vi "day 11 task 2.vi"() -> ()   [LabVIEW 2019]
uses:
  <userlib>/_OpenG.lib/array/array.llb/Search 1D Array (I32)__ogtk.vi
panel:
  out "Monkeys":T1(array[cluster])
  out "Array":T1(array[cluster])
  out "level of monkey business":u64
  out "Amount of inspections by each monkey":u64[](array[numeric])
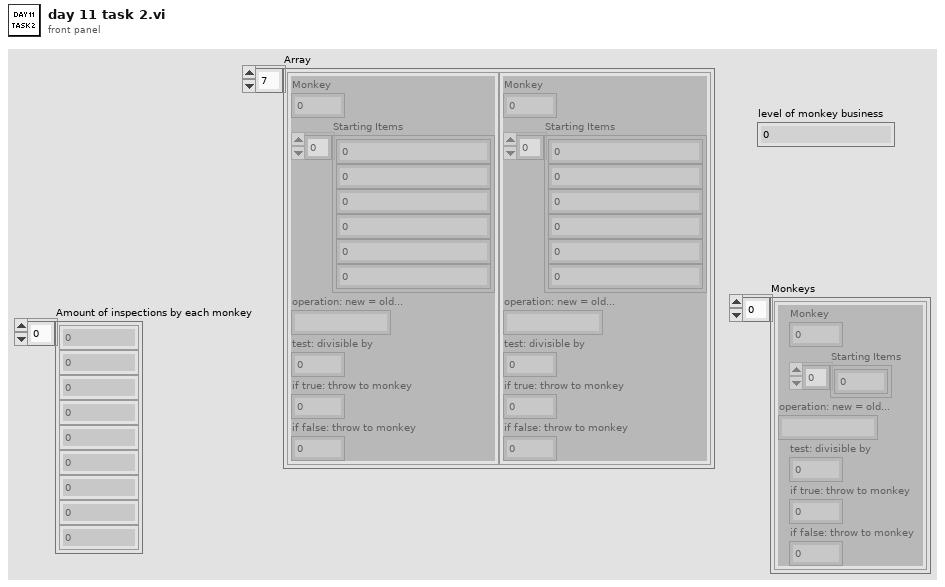
[diagram p1: front panel]
types:
  T1 = cluster{"Monkey":i32, "Starting Items":u64[], "operation: new = old...":string, "test: divisible by":u64, "if true: throw to monkey":i32, "if false: throw to monkey":i32}[]
  T2 = cluster{"Monkey":i32, "Starting Items":u64[], "operation: new = old...":string, "test: divisible by":u64, "if true: throw to monkey":i32, "if false: throw to monkey":i32}
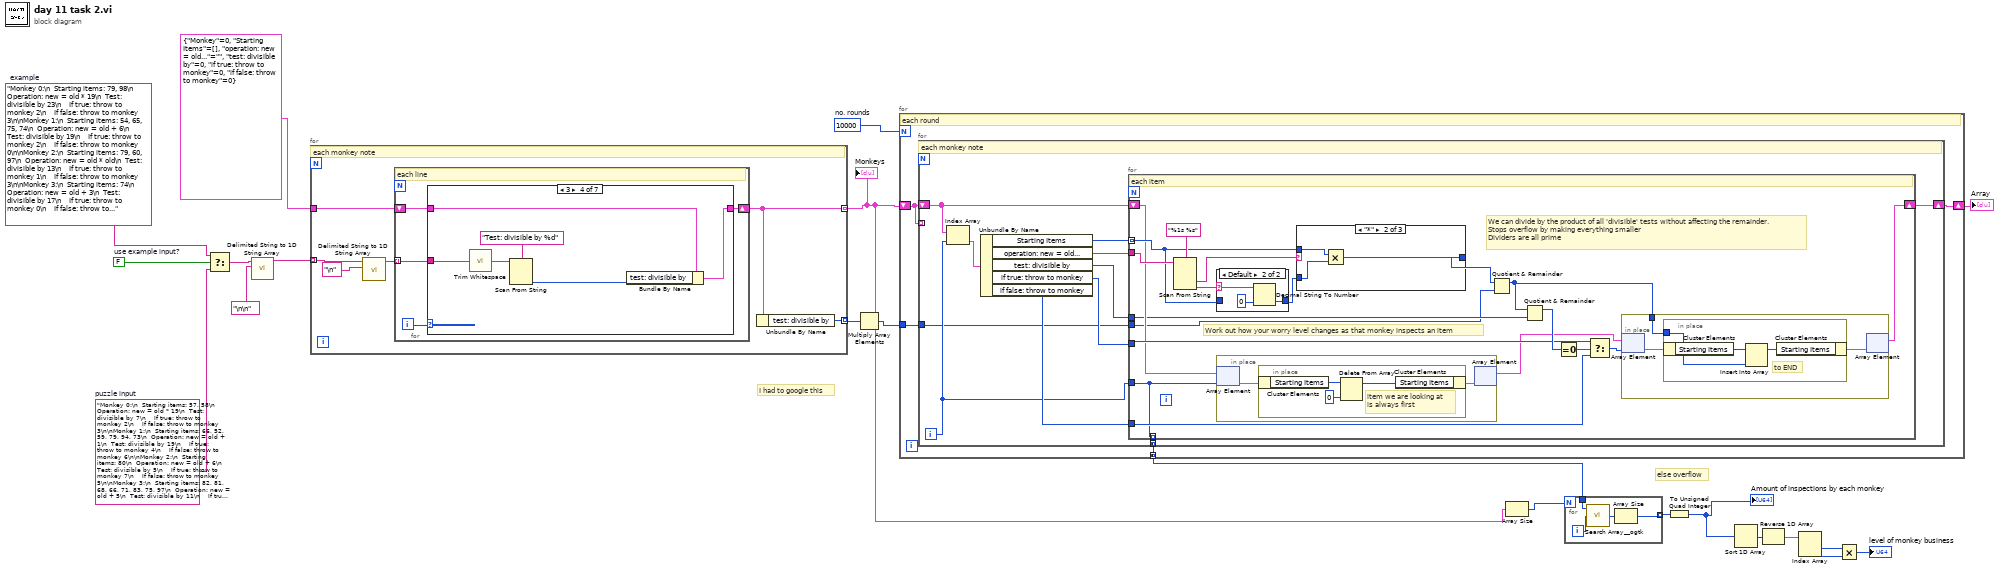
[diagram p0: block diagram]
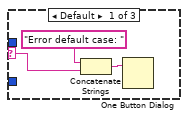
[diagram p3: hidden frame]
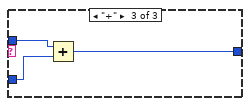
[diagram p4: hidden frame]
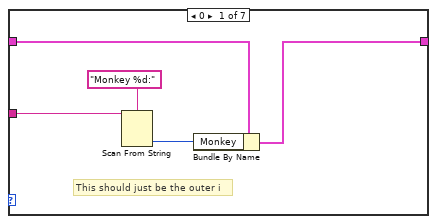
[diagram p5: hidden frame]
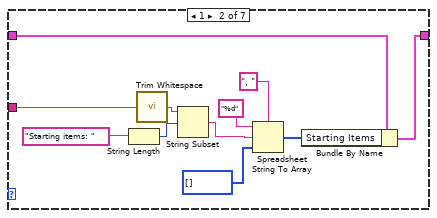
[diagram p6: hidden frame]
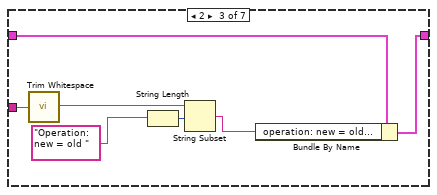
[diagram p7: hidden frame]
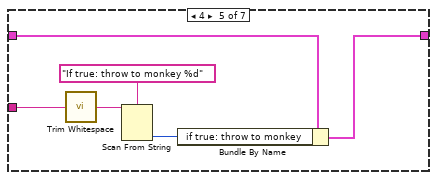
[diagram p8: hidden frame]
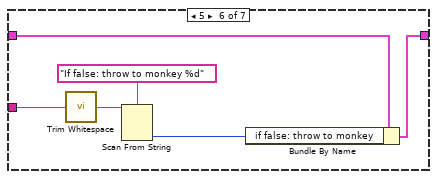
[diagram p9: hidden frame]
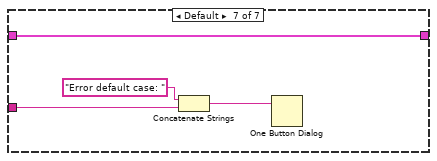
[diagram p10: hidden frame]
diagram:
  w14 = 10000  # no. rounds
  w19 = "Monkey 0:\n  Starting items: 79, 98\n  Operation: new = old * 19\n  Test: divisible by 23\n    If true: throw to monkey 2\n    If false: throw to monkey 3\n\nMonkey 1:\n  Starting items: 54, 65, 75, 74\n  Operation: new = old + 6\n  Test: divisible by 19\n    If true: throw to monkey 2\n    If false: throw to monkey 0\n\nMonkey 2:\n  Starting items: 79, 60, 97\n  Operation: new = old * old\n  Test: divisible by 13\n    If true: throw to monkey 1\n    If false: throw to monkey 3\n\nMonkey 3:\n  Starting items: 74\n  Operation: new = old + 3\n  Test: divisible by 17\n    If true: throw to monkey 0\n    If false: throw to monkey 1"  # example
  w20 = FALSE  # use example input?
  w21 = "Monkey 0:\n  Starting items: 57, 58\n  Operation: new = old * 19\n  Test: divisible by 7\n    If true: throw to monkey 2\n    If false: throw to monkey 3\n\nMonkey 1:\n  Starting items: 66, 52, 59, 79, 94, 73\n  Operation: new = old + 1\n  Test: divisible by 19\n    If true: throw to monkey 4\n    If false: throw to monkey 6\n\nMonkey 2:\n  Starting items: 80\n  Operation: new = old + 6\n  Test: divisible by 5\n    If true: throw to monkey 7\n    If false: throw to monkey 5\n\nMonkey 3:\n  Starting items: 82, 81, 68, 66, 71, 83, 75, 97\n  Operation: new = old + 5\n  Test: divisible by 11\n    If true: throw to monkey 5\n    If false: throw to monkey 2\n\nMonkey 4:\n  Starting items: 55, 52, 67, 70, 69, 94, 90\n  Operation: new = old * old\n  Test: divisible by 17\n    If true: throw to monkey 0\n    If false: throw to monkey 3\n\nMonkey 5:\n  Starting items: 69, 85, 89, 91\n  Operation: new = old + 7\n  Test: divisible by 13\n    If true: throw to monkey 1\n    If false: throw to monkey 7\n\nMonkey 6:\n  Starting items: 75, 53, 73, 52, 75\n  Operation: new = old * 7\n  Test: divisible by 2\n    If true: throw to monkey 0\n    If false: throw to monkey 4\n\nMonkey 7:\n  Starting items: 94, 60, 79\n  Operation: new = old + 2\n  Test: divisible by 3\n    If true: throw to monkey 1\n    If false: throw to monkey 6"  # puzzle input
  # "else overflow"
  # "I had to google this"
  n1 = Select(t=w19, s=w20, f=w21) -> (s? t:f=w18:string)
  n2 = call <vilib>:"Delimited String to 1D String Array.vi"("delimiter"="\n\n" ("regular expression"), "delimited string"=w18) -> ("string array"=w16:string[])  [unwired: 9 in]
  n3 = for {
    tunnel: w16 -> [w27] mode=indexing
    tunnel: T2 {"Monkey"=0, "Starting Items"=[], "operation: new = old..."="", "test: divisible by"=0, "if true: throw to monkey"=0, "if false: throw to monkey"=0} -> [w26]
    tunnel: [w23] -> w12 mode=indexing
    tunnel: [w22] -> w4 mode=indexing
    # "each monkey note"
    n4 = call <vilib>:"Delimited String to 1D String Array.vi"("delimiter"="\n", "delimited string"=w27) -> ("string array"=w25:string[])  [unwired: 9 in]
    n5 = for {
      tunnel: w25 -> [w30] mode=indexing
      shift-right: [w29] -> w23
      shift-left: w26 -> [w28]
      i -> [w31]
      # "each line"
      n6 = case shown="3" w31 {
        tunnel: w30 -> [w36 w44 w54 w58 w64 w70 w74]
        tunnel: [w34 w41 w52 w55 w61 w67 w73] -> w29
        tunnel: w28 -> [w33 w42 w53 w56 w62 w69 w73]
        frame 0 {
          # "This should just be the outer i"
          n7 = Scan From String(format string="Monkey %d:", input string=w36) -> (output 1=w32:i32)  [unwired: 3 in, 3 out]
          n8 = Bundle By Name(cluster=w33, "Monkey"=w32) -> (w34:T2)
        }
        frame 1 {
          n9 = String Length(string="Starting items: " ("format string")) -> (length=w38:i32)
          n10 = call <vilib>:"Trim Whitespace.vi"("string"=w44) -> ("trimmed string"=w37:string)  [unwired: 1 in]
          n11 = String Subset(string=w37, offset (0)=w38) -> (substring=w40:string)  [unwired: 1 in]
          n12 = Spreadsheet String To Array(delimiter (Tab)=", ", format string="%d", spreadsheet string=w40, array type (2D Dbl)=u64[] []) -> (array=w43:u64[])
          n13 = Bundle By Name(cluster=w42, "Starting Items"=w43) -> (w41:T2)
        }
        frame 2 {
          n14 = call <vilib>:"Trim Whitespace.vi"("string"=w54) -> ("trimmed string"=w50:string)  [unwired: 1 in]
          n15 = String Length(string="Operation: new = old " ("format string")) -> (length=w48:i32)
          n16 = String Subset(string=w50, offset (0)=w48) -> (substring=w51:string)  [unwired: 1 in]
          n17 = Bundle By Name(cluster=w53, "operation: new = old..."=w51) -> (w52:T2)
        }
        frame 3 {
          n18 = call <vilib>:"Trim Whitespace.vi"("string"=w58) -> ("trimmed string"=w59:string)  [unwired: 1 in]
          n19 = Scan From String(format string="Test: divisible by %d", input string=w59) -> (output 1=w57:i32)  [unwired: 3 in, 3 out]
          n20 = Bundle By Name(cluster=w56, "test: divisible by"=w57) -> (w55:T2)
        }
        frame 4 {
          n21 = call <vilib>:"Trim Whitespace.vi"("string"=w64) -> ("trimmed string"=w65:string)  [unwired: 1 in]
          n22 = Scan From String(format string="If true: throw to monkey %d", input string=w65) -> (output 1=w63:i32)  [unwired: 3 in, 3 out]
          n23 = Bundle By Name(cluster=w62, "if true: throw to monkey"=w63) -> (w61:T2)
        }
        frame 5 {
          n24 = call <vilib>:"Trim Whitespace.vi"("string"=w70) -> ("trimmed string"=w71:string)  [unwired: 1 in]
          n25 = Scan From String(format string="If false: throw to monkey %d", input string=w71) -> (output 1=w68:i32)  [unwired: 3 in, 3 out]
          n26 = Bundle By Name(cluster=w69, "if false: throw to monkey"=w68) -> (w67:T2)
        }
        frame Default {
          n27 = Concatenate Strings("Error default case: " ("message"), w74) -> (w75:string)
          n28 = One Button Dialog(message=w75) -> ()  [unwired: 1 in, 1 out]
        }
      }
    }
    n29 = Unbundle By Name(w23) -> ("test: divisible by"=w22:u64)
  }
  "Monkeys" <- w12
  n30 = Multiply Array Elements(1:w4) -> (0:w3:u64)
  n31 = for {
    N: w14 -> [_]
    shift-right: [w80] -> w5
    shift-left: w12 -> [w79]
    tunnel: [w78] -> w11 mode=concatenating
    tunnel: w3 -> [w77]
    # "each round"
    n32 = for {
      shift-right: [w87] -> w80
      shift-left: w79 -> [w86]
      tunnel: w79 -> [_] mode=indexing
      tunnel: [w82] -> w78 mode=concatenating
      tunnel: w77 -> [w81]
      i -> [w83]
      # "each monkey note"
      n33 = Index Array(array=w86, index=w83) -> (element=w90:T2)
      n34 = Unbundle By Name(w90) -> ("Starting Items"=w91:u64[], "operation: new = old..."=w89:string, "test: divisible by"=w88:u64, "if true: throw to monkey"=w85:i32, "if false: throw to monkey"=w84:i32)
      n35 = for {
        tunnel: w91 -> [w105] mode=indexing
        tunnel: w89 -> [w110]
        tunnel: w88 -> [w95]
        shift-right: [w97] -> w87
        shift-left: w86 -> [w99]
        tunnel: w85 -> [w102]
        tunnel: w84 -> [w101]
        tunnel: w83 -> [w96]
        tunnel: [w96] -> w82 mode=indexing
        tunnel: w81 -> [w93]
        # "We can divide by the product of all 'divisible' tests without affecting the remainder.\nStops overflow by making everything smaller\nDividers are all prime"
        # "Work out how your worry level changes as that monkey inspects an item"
        # "each item"
        n36 = Scan From String(format string="%1s %s", input string=w110) -> (output 1=w108:string, output 2=w107:string)  [unwired: 4 in, 3 out]
        n37 = case shown="Default" w107 {
          selector: w107 -> [_ w125]
          tunnel: [w122 w124] -> w106
          tunnel: w105 -> [w122 _]
          frame "old" {
          }
          frame Default {
            n38 = Decimal String To Number(string=w125, default (0L)=u64 0) -> (number=w124:u64)  [unwired: 1 in, 1 out]
          }
        }
        n39 = in-place {
          n40 = in-place-array #1(w99, w96) -> (w118:T2)
          n41 = in-place {
            # "item we are looking at \nis always first"
            n42 = in-place-cluster #2(w118) -> ("Starting Items"=w120:u64[])
            n43 = Delete From Array(array=w120, index=0) -> (array with subset deleted=w121:u64[])  [unwired: 1 in, 1 out]
            n44 = in-place-cluster #2("Starting Items"=w121) -> (w117:T2)
          }
          n45 = in-place-array #1(w117) -> (w98:T1)  [unwired: 1 out]
        }
        n46 = case shown="\"*\"" w108 {
          selector: w108 -> [w126 _ _]
          tunnel: w106 -> [_ w130 w134]
          tunnel: w105 -> [_ w131 w133]
          tunnel: [_ w129 w132] -> w94
          frame Default {
            n47 = Concatenate Strings("Error default case: " ("message"), w126) -> (w128:string)
            n48 = One Button Dialog(message=w128) -> ()  [unwired: 1 in, 1 out]
          }
          frame "*" {
            n49 = Multiply(x=w131, y=w130) -> (x*y=w129:u64)
          }
          frame "+" {
            n50 = Add(x=w133, y=w134) -> (x+y=w132:u64)
          }
        }
        n51 = Quotient & Remainder(x=w94, y=w93) -> (x-y*floor(x/y)=w92:u64)  [unwired: 1 out]
        n52 = Quotient & Remainder(x=w92, y=w95) -> (x-y*floor(x/y)=w104:u64)  [unwired: 1 out]
        n53 = Equal To 0?(x=w104) -> (x = 0?=w103:bool)
        n54 = Select(t=w102, s=w103, f=w101) -> (s? t:f=w100:i32)
        n55 = in-place {
          in-place-border: w92 -> [w113]
          n56 = in-place-array #3(w98, w100) -> (w111:T2)
          n57 = in-place {
            in-place-border: w113 -> [w115]
            # "to END"
            n58 = in-place-cluster #4(w111) -> ("Starting Items"=w114:u64[])
            n59 = Insert Into Array(array=w114, new element=w115) -> (w116:u64[])  [unwired: 1 in]
            n60 = in-place-cluster #4("Starting Items"=w116) -> (w112:T2)
          }
          n61 = in-place-array #3(w112) -> (w97:T1)  [unwired: 1 out]
        }
      }
    }
  }
  "Array" <- w5
  n62 = Array Size(array=w12) -> (size(s)=w13:i32)
  n63 = for {
    N: w13 -> [_]
    tunnel: w11 -> [w138]
    tunnel: [w135] -> w2 mode=indexing
    i -> [w137]
    n64 = call-poly <userlib>:"Search Array__ogtk.vi"("Array"=w138, "Element Data"=w137) -> ("Indices of Elements"=w136:i32[])  [unwired: 7 in]
    n65 = Array Size(array=w136) -> (size(s)=w135:i32)
  }
  n66 = To Unsigned Quad Integer(1:w2) -> (0:w1:u64[])
  "Amount of inspections by each monkey" <- w1
  n67 = Sort 1D Array(array=w1) -> (sorted array=w7:u64[])
  n68 = Reverse 1D Array(array=w7) -> (reversed array=w6:u64[])
  n69 = Index Array(array=w6) -> (element #1=w10:u64, element #2=w9:u64)  [unwired: 2 in]
  n70 = Multiply(x=w10, y=w9) -> (x*y=→"level of monkey business":u64)
